vi "系统参数设置.vi"(8 "错误输入":errorcluster caption="错误常量") -> (0 "错误输出":errorcluster caption="错误常量")   [LabVIEW 2018]
uses:
  gbl.vi
panel:
  in  "更新显示":bool
  in  "加载配置文件":bool
  in  "设置完成":bool
  in  "外同步极性":u8(ring) items=["负极", "正极性"]
  in  "数据传输率/Hz":sgl=1.0 caption="数值输入控件"
  in  "采样平均次数":u8=1 caption="数值输入控件"
  in  "自动增益百分比":u16=100 caption="数值输入控件" max=100 step=1
  in  "自动增益":u8(ring) items=["关", "开"]
  in  "检测范围":sgl=20.0 caption="数值输入控件"
  in  "dB码":u16=30 caption="数值输入控件"
  in  "零位延时/us":dbl caption="数值输入控件" min=0.0 max=50.0 step=0.01
  in  "采样深度":u16=4096 caption="数值输入控件" min=1 max=4096 step=1
  in  "脉冲宽度/ns":u32=70 caption="数值输入控件" min=30 max=1000 step=1
  in  "重复频率/Hz":sgl=10.0 caption="数值输入控件" min=10 max=10000 step=1
  in  "发射电压/V":u32=300 caption="数值输入控件" min=20 max=300 step=1
  in  "检波模式":u8(ring)=3 items=["全检波", "正检波", "负检波", "射频"]
  in  "触发模式":u8(ring) items=["定时模式", "编码器模式", "外同步信号"]
  in  "阻抗匹配":u8(ring) items=["50欧姆", "500欧姆"]
  in  "收发模式":u8(ring) items=["自发自收", "单发单收", "穿透"]
  in  "通道":u8(ring) items=["通道一", "通道二", "通道三", "通道四"]
  # "硬件参数设置"
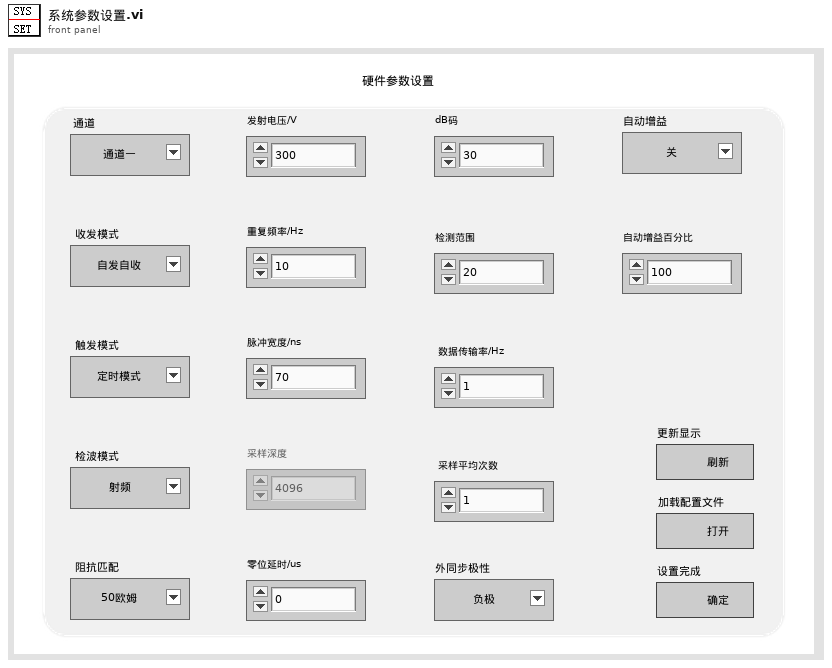
[diagram p1: front panel]
types:
  T1 = enum8{"Enabled", "Disabled", "Disabled and Grayed Out"}
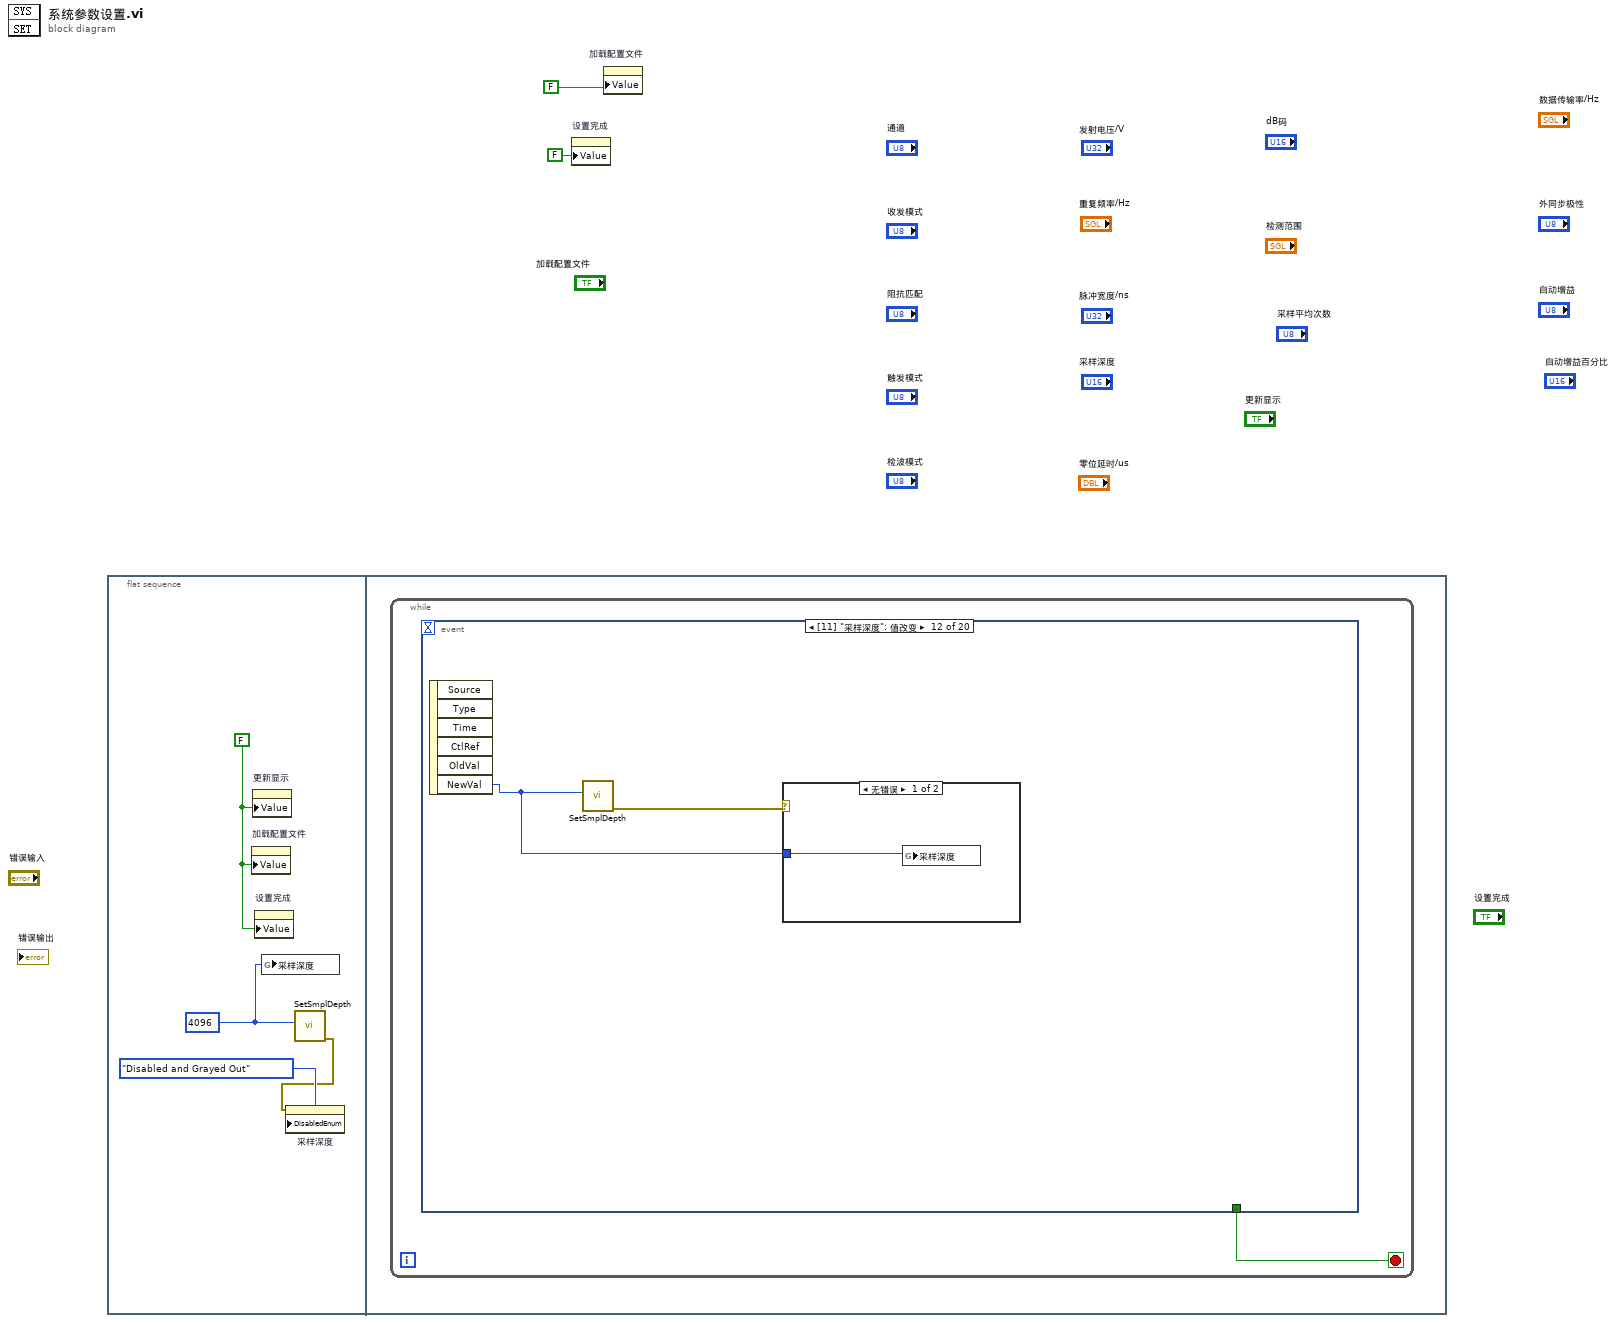
[diagram p0: block diagram]
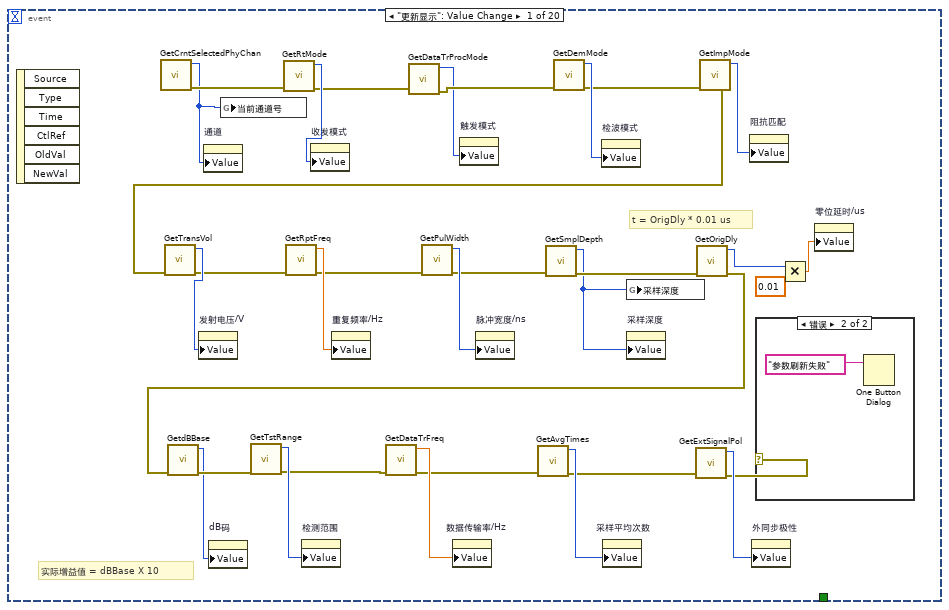
[diagram p2: hidden frame]
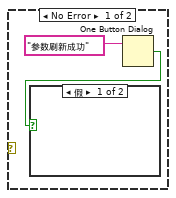
[diagram p3: hidden frame]
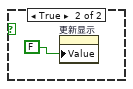
[diagram p4: hidden frame]
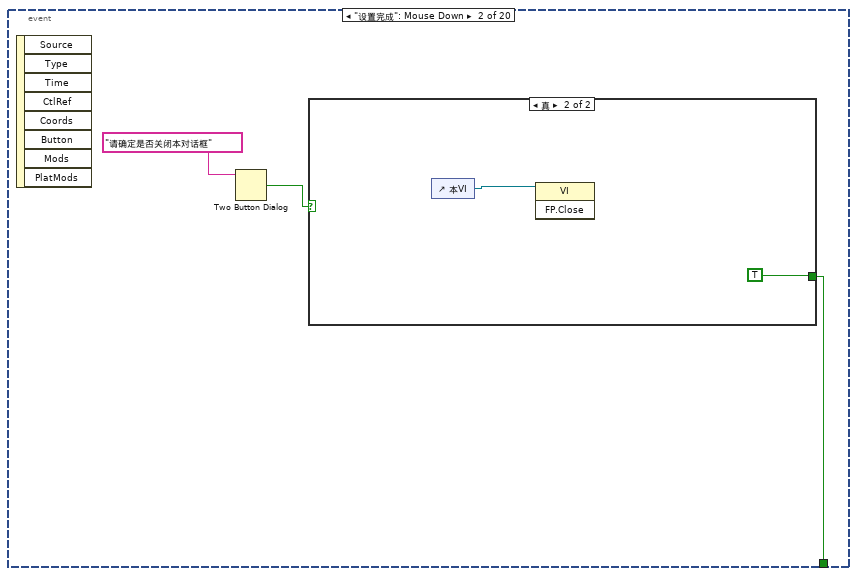
[diagram p5: hidden frame]
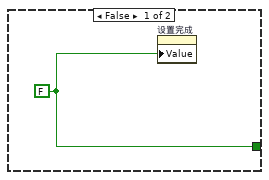
[diagram p6: hidden frame]
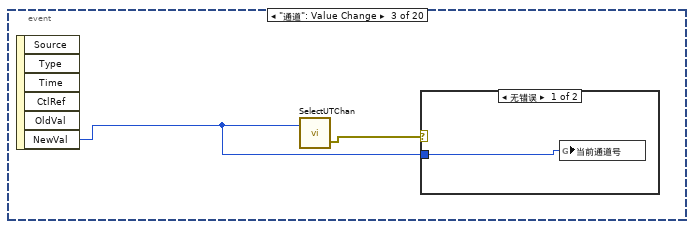
[diagram p7: hidden frame]
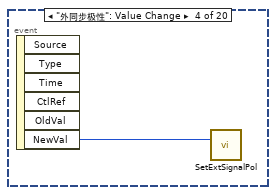
[diagram p9: hidden frame]
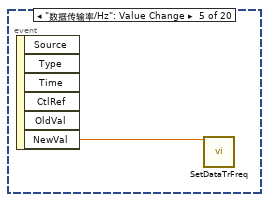
[diagram p10: hidden frame]
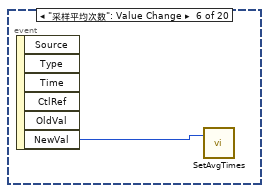
[diagram p11: hidden frame]
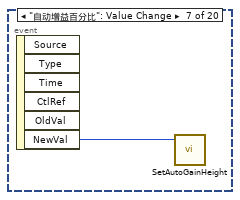
[diagram p12: hidden frame]
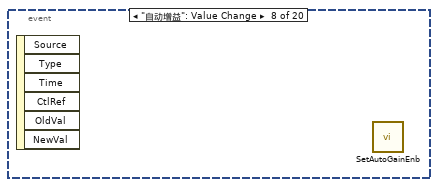
[diagram p13: hidden frame]
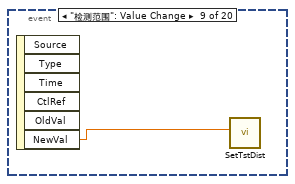
[diagram p14: hidden frame]
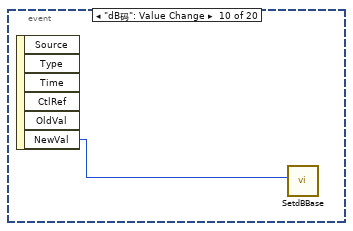
[diagram p15: hidden frame]
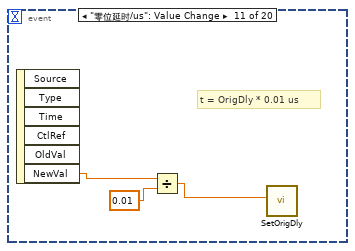
[diagram p16: hidden frame]
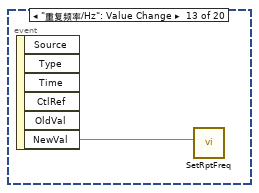
[diagram p18: hidden frame]
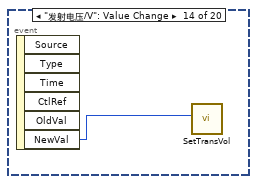
[diagram p19: hidden frame]
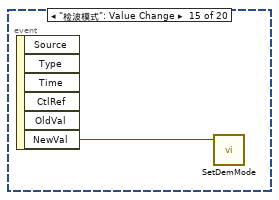
[diagram p20: hidden frame]
diagram:
  n1 = flat-sequence {
    frame #0 {
      w3 = u16 4096 ("采样深度")
      w6 = FALSE
      n2 = property on="加载配置文件" class="Bool (严格)"("Value"=w6) -> ()  [unwired: 2 in, 2 out]
      n3 = property on="更新显示" class="Bool (严格)"("Value"=w6) -> ()  [unwired: 2 in, 2 out]
      n4 = property on="设置完成" class="Bool (严格)"("Value"=w6) -> ()  [unwired: 2 in, 2 out]
      n5 = global write "gbl.vi" "采样深度"(w3) -> ()
      n6 = call "SetSmplDepth.vi"("采样深度"=w3) -> ("错误输出"=w4:errorcluster)  [unwired: 10 in]
      n7 = property on="采样深度" class="DigNum (严格)"(error in=w4, "DisabledEnum"=T1."Disabled and Grayed Out" ("禁用")) -> ()  [unwired: 1 in, 2 out]
    }
    frame #1 {
      n8 = while {
        stop <- w7 stop-if-true
        n9 = event shown="[11] \"采样深度\": 值改变" {
          selector: _ -> [_ _ _ _ _ _ _ _ _ _ _ _ _ _ _ _ _ _ _ _]
          dyn-events: _ -> [_ _ _ _ _ _ _ _ _ _ _ _ _ _ _ _ _ _ _ _]
          timeout: _ -> [_ _ _ _ _ _ _ _ _ _ _ _ _ _ _ _ _ _ _ _]
          tunnel: [_ w44 _ _ _ _ _ _ _ _ _ _ _ _ _ _ _ _ _ _] -> w7
          event "更新显示": Value Change {
            # "实际增益值 = dBBase X 10"
            # "t = OrigDly * 0.01 us"
            n10 = event-data() -> ()  [unwired: 1 in, 6 out]
            n11 = call "GetCrntSelectedPhyChan.vi"() -> ("错误输出"=w38:errorcluster, "返回值"=w8:u8)  [unwired: 10 in]
            n12 = property on="通道" class="Ring (严格)"("Value"=w8) -> ()  [unwired: 2 in, 2 out]
            n13 = global write "gbl.vi" "当前通道号"(w8) -> ()
            n14 = call "GetRtMode.vi"("错误输入（无错误）"=w38) -> ("错误输出"=w12:errorcluster, "返回值"=w39:u8)  [unwired: 9 in]
            n15 = property on="收发模式" class="Ring (严格)"("Value"=w39) -> ()  [unwired: 2 in, 2 out]
            n16 = call "GetDataTrProcMode.vi"("错误输入（无错误）"=w12) -> ("错误输出"=w11:errorcluster, "返回值"=w10:u8)  [unwired: 9 in]
            n17 = property on="触发模式" class="Ring (严格)"("Value"=w10) -> ()  [unwired: 2 in, 2 out]
            n18 = call "GetDemMode.vi"("错误输入（无错误）"=w11) -> ("错误输出"=w36:errorcluster, "返回值"=w37:u8)  [unwired: 9 in]
            n19 = property on="检波模式" class="Ring (严格)"("Value"=w37) -> ()  [unwired: 2 in, 2 out]
            n20 = call "GetImpMode.vi"("错误输入（无错误）"=w36) -> ("错误输出"=w34:errorcluster, "返回值"=w35:u8)  [unwired: 9 in]
            n21 = call "GetTransVol.vi"("错误输入（无错误）"=w34) -> ("错误输出"=w32:errorcluster, "返回值"=w33:u32)  [unwired: 9 in]
            n22 = property on="发射电压/V" class="DigNum (严格)"("Value"=w33) -> ()  [unwired: 2 in, 2 out]
            n23 = call "GetRptFreq.vi"("错误输入（无错误）"=w32) -> ("错误输出"=w30:errorcluster, "返回值"=w31:sgl)  [unwired: 9 in]
            n24 = property on="重复频率/Hz" class="DigNum (严格)"("Value"=w31) -> ()  [unwired: 2 in, 2 out]
            n25 = call "GetPulWidth.vi"("错误输入（无错误）"=w30) -> ("错误输出"=w28:errorcluster, "返回值"=w29:u32)  [unwired: 9 in]
            n26 = property on="脉冲宽度/ns" class="DigNum (严格)"("Value"=w29) -> ()  [unwired: 2 in, 2 out]
            n27 = call "GetSmplDepth.vi"("错误输入（无错误）"=w28) -> ("错误输出"=w27:errorcluster, "返回值"=w13:u16)  [unwired: 9 in]
            n28 = global write "gbl.vi" "采样深度"(w13) -> ()
            n29 = property on="采样深度" class="DigNum (严格)"("Value"=w13) -> ()  [unwired: 2 in, 2 out]
            n30 = call "GetOrigDly.vi"("错误输入（无错误）"=w27) -> ("错误输出"=w26:errorcluster, "返回值"=w25:u32)  [unwired: 9 in]
            n31 = call "GetdBBase.vi"("错误输入（无错误）"=w26) -> ("错误输出"=w22:errorcluster, "返回值"=w9:u16)  [unwired: 9 in]
            n32 = property on="dB码" class="DigNum (严格)"("Value"=w9) -> ()  [unwired: 2 in, 2 out]
            n33 = call "GetTstRange.vi"("错误输入（无错误）"=w22) -> ("错误输出"=w19:errorcluster, "返回值"=w21:u16)  [unwired: 9 in]
            n34 = property on="检测范围" class="DigNum (严格)"("Value"=w21) -> ()  [unwired: 2 in, 2 out]
            n35 = call "GetDataTrFreq.vi"("错误输入（无错误）"=w19) -> ("错误输出"=w18:errorcluster, "返回值"=w20:sgl)  [unwired: 9 in]
            n36 = property on="数据传输率/Hz" class="DigNum (严格)"("Value"=w20) -> ()  [unwired: 2 in, 2 out]
            n37 = call "GetAvgTimes.vi"("错误输入（无错误）"=w18) -> ("错误输出"=w16:errorcluster, "当前通道采样平均次数"=w17:u8)  [unwired: 9 in]
            n38 = property on="采样平均次数" class="DigNum (严格)"("Value"=w17) -> ()  [unwired: 2 in, 2 out]
            n39 = call "GetExtSignalPol.vi"("错误输入（无错误）"=w16) -> ("错误输出"=w14:errorcluster, "返回值"=w15:u8)  [unwired: 9 in]
            n40 = property on="阻抗匹配" class="Ring (严格)"("Value"=w35) -> ()  [unwired: 2 in, 2 out]
            n41 = property on="外同步极性" class="Ring (严格)"("Value"=w15) -> ()  [unwired: 2 in, 2 out]
            n42 = case shown="错误" w14 {
              frame No Error {
                n43 = One Button Dialog(message="参数刷新成功" ("消息")) -> (true=w40:bool)  [unwired: 1 in]
                n44 = case shown="假" w40 {
                  frame False {
                  }
                  frame True {
                    n45 = property on="更新显示" class="Bool (严格)"("Value"=FALSE) -> ()  [unwired: 2 in, 2 out]
                  }
                }
              }
              frame Error {
                n46 = One Button Dialog(message="参数刷新失败" ("消息")) -> ()  [unwired: 1 in, 1 out]
              }
            }
            n47 = Multiply(x=w25, y=0.01) -> (x*y=w24:dbl)
            n48 = property on="零位延时/us" class="DigNum (严格)"("Value"=w24) -> ()  [unwired: 2 in, 2 out]
          }
          event "设置完成": Mouse Down {
            n49 = event-data() -> ()  [unwired: 1 in, 8 out]
            n50 = Two Button Dialog(message="请确定是否关闭本对话框" ("消息")) -> (T button?=w45:bool)  [unwired: 2 in]
            n51 = case shown="真" w45 {
              tunnel: [w47 TRUE] -> w44
              frame False {
                w47 = FALSE
                n52 = property on="设置完成" class="Bool (严格)"("Value"=w47) -> ()  [unwired: 2 in, 2 out]
              }
              frame True {
                n53 = control-ref of="本VI"() -> (w49:refnum<vi>)
                n54 = invoke class="VI" method="FP.Close"(reference=w49) -> ()  [unwired: 2 in, 3 out]
              }
            }
          }
          event "通道": Value Change {
            n55 = event-data() -> ("NewVal"=w50:u8)  [unwired: 1 in, 5 out]
            n56 = call "SelectUTChan.vi"("指定的通道号"=w50) -> ("错误输出"=w51:errorcluster)  [unwired: 2 in]
            n57 = case shown="无错误" w51 {
              tunnel: w50 -> [w52 _]
              frame No Error {
                n58 = global write "gbl.vi" "当前通道号"(w52) -> ()
              }
              frame Error {
              }
            }
          }
          event "外同步极性": Value Change {
            n59 = event-data() -> ("NewVal"=w53:u8)  [unwired: 1 in, 5 out]
            n60 = call "SetExtSignalPol.vi"("外同步信号极性"=w53) -> ()  [unwired: 10 in, 1 out]
          }
          event "数据传输率/Hz": Value Change {
            n61 = event-data() -> ("NewVal"=w54:sgl)  [unwired: 1 in, 5 out]
            n62 = call "SetDataTrFreq.vi"("数据传输率"=w54) -> ()  [unwired: 10 in, 1 out]
          }
          event "采样平均次数": Value Change {
            n63 = event-data() -> ("NewVal"=w55:u8)  [unwired: 1 in, 5 out]
            n64 = call "SetAvgTimes.vi"("采样平均次数"=w55) -> ()  [unwired: 2 in, 1 out]
          }
          event "自动增益百分比": Value Change {
            n65 = event-data() -> ("NewVal"=w56:u16)  [unwired: 1 in, 5 out]
            n66 = call "SetAutoGainHeight.vi"("自动增益高度百分比"=w56) -> ()  [unwired: 2 in, 1 out]
          }
          event "自动增益": Value Change {
            n67 = event-data() -> ()  [unwired: 1 in, 6 out]
            n68 = call "SetAutoGainEnb.vi"() -> ()  [unwired: 11 in, 1 out]
          }
          event "检测范围": Value Change {
            n69 = event-data() -> ("NewVal"=w57:sgl)  [unwired: 1 in, 5 out]
            n70 = call "SetTstDist.vi"("检测范围"=w57) -> ()  [unwired: 8 in, 1 out]
          }
          event "dB码": Value Change {
            n71 = event-data() -> ("NewVal"=w58:u16)  [unwired: 1 in, 5 out]
            n72 = call "SetdBBase.vi"("增益值索引"=w58) -> ()  [unwired: 10 in, 1 out]
          }
          event "零位延时/us": Value Change {
            # "t = OrigDly * 0.01 us"
            n73 = event-data() -> ("NewVal"=w61:dbl)  [unwired: 1 in, 5 out]
            n74 = Divide(x=w61, y=0.01) -> (x/y=w59:dbl)
            n75 = call "SetOrigDly.vi"("OrigDly"=w59) -> ()  [unwired: 10 in, 1 out]
          }
          event "采样深度": Value Change {
            n76 = event-data() -> ("NewVal"=w62:u16)  [unwired: 1 in, 5 out]
            n77 = call "SetSmplDepth.vi"("采样深度"=w62) -> ("错误输出"=w63:errorcluster)  [unwired: 10 in]
            n78 = case shown="无错误" w63 {
              tunnel: w62 -> [w64 _]
              frame No Error {
                n79 = global write "gbl.vi" "采样深度"(w64) -> ()
              }
              frame Error {
              }
            }
          }
          event "重复频率/Hz": Value Change {
            n80 = event-data() -> ("NewVal"=w65:sgl)  [unwired: 1 in, 5 out]
            n81 = call "SetRptFreq.vi"("采样重复频率"=w65) -> ()  [unwired: 10 in, 1 out]
          }
          event "发射电压/V": Value Change {
            n82 = event-data() -> ("NewVal"=w66:u32)  [unwired: 1 in, 5 out]
            n83 = call "SetTransVol.vi"("发射电压"=w66) -> ()  [unwired: 10 in, 1 out]
          }
          event "检波模式": Value Change {
            n84 = event-data() -> ("NewVal"=w67:u8)  [unwired: 1 in, 5 out]
            n85 = call "SetDemMode.vi"("检波模式索引值"=w67) -> ()  [unwired: 10 in, 1 out]
          }
          event "触发模式": Value Change {
            n86 = event-data() -> ("NewVal"=w68:u8)  [unwired: 1 in, 5 out]
            n87 = call "SetDataTrProcMode.vi"("数据传输模式"=w68) -> ()  [unwired: 10 in, 1 out]
          }
          event "阻抗匹配": Value Change {
            n88 = event-data() -> ("NewVal"=w69:u8)  [unwired: 1 in, 5 out]
            n89 = call "SetImpMode.vi"("阻抗模式"=w69) -> ()  [unwired: 10 in, 1 out]
          }
          event "收发模式": Value Change {
            n90 = event-data() -> ("NewVal"=w70:u8)  [unwired: 1 in, 5 out]
            n91 = call "SetRtMode.vi"("收发模式"=w70) -> ()  [unwired: 10 in, 1 out]
          }
          event "脉冲宽度/ns": Value Change {
            n92 = event-data() -> ("NewVal"=w71:u32)  [unwired: 1 in, 5 out]
            n93 = call "SetPulWidth.vi"("采样脉冲宽度"=w71) -> ()  [unwired: 10 in, 1 out]
          }
          event "加载配置文件": Value Change {
            n94 = event-data() -> ()  [unwired: 1 in, 6 out]
            n95 = flat-sequence {
              frame #0 {
                n96 = call "LoadUTCraftFile.vi"() -> ()  [unwired: 11 in, 1 out]
              }
              frame #1 {
                n97 = property on="加载配置文件" class="Bool (严格)"("Value"=FALSE) -> ()  [unwired: 2 in, 2 out]
              }
            }
          }
        }
      }
    }
  }
  n98 = property on="设置完成" class="Bool (严格)"("Value"=FALSE) -> ()  [unwired: 2 in, 2 out]
  n99 = property on="加载配置文件" class="Bool (严格)"("Value"=FALSE) -> ()  [unwired: 2 in, 2 out]
